vi "diffpsk.vi"() -> ()   [LabVIEW 2014]
panel:
  out "decoded\n data 2":bool[](array[boolean])
  out "demodulated output":dynamicdata(graph)
  out "Waveform DPSK":dynamicdata(graph)
  out "encoded data":bool[](array[boolean])
  in  "binary data":bool[](array[boolean])
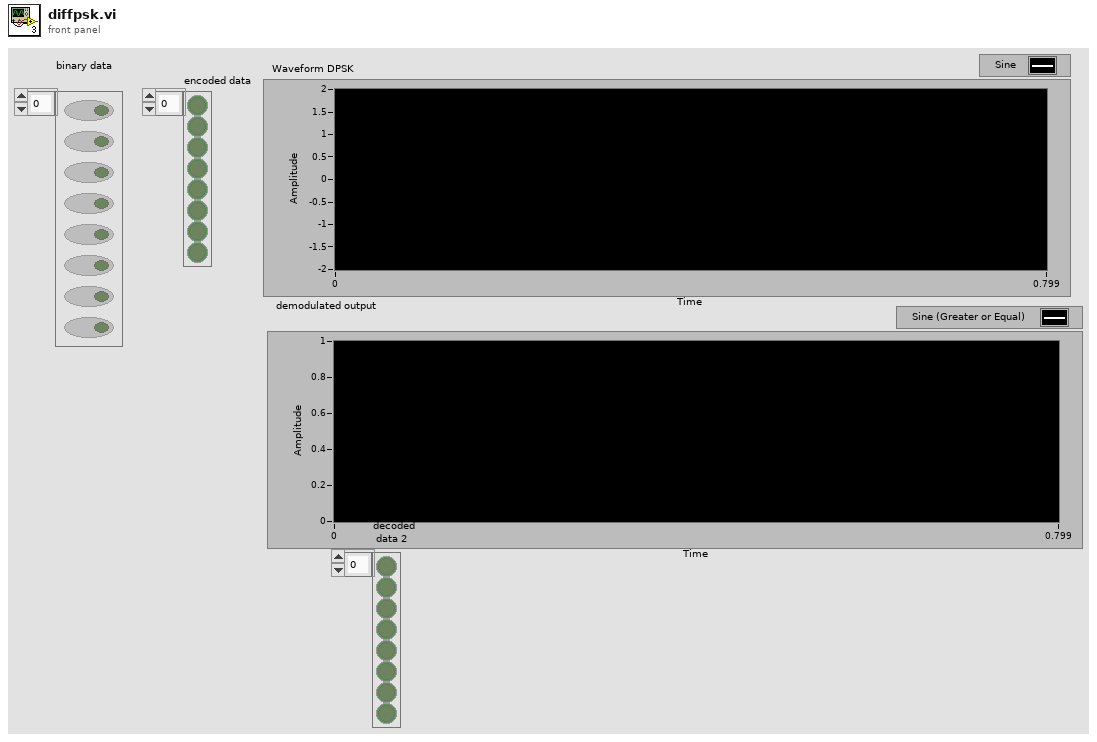
[diagram p1: front panel]
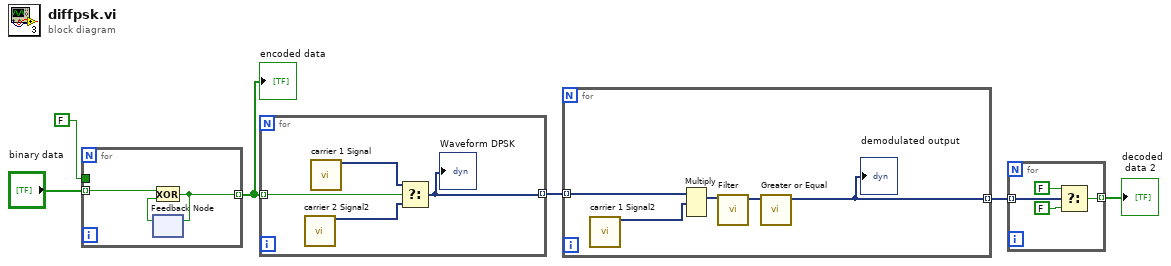
[diagram p0: block diagram]
diagram:
  n1 = for {
    tunnel: "binary data" -> [w9] mode=indexing
    tunnel: FALSE -> [_]
    tunnel: [w7] -> w4 mode=indexing
    n2 = feedback #1() -> (w8:bool)  [unwired: 1 in]
    n3 = Exclusive Or(1:w8, 2:w9) -> (0:w7:bool)
    n4 = feedback-in #1(w7) -> ()
  }
  "encoded data" <- w4
  n5 = for {
    tunnel: w4 -> [w11] mode=indexing
    tunnel: [w10] -> w3 mode=indexing
    n6 = call "carrier 2 Signal2"() -> ("Sine"=w12:dynamicdata)  [unwired: 14 in, 1 out]
    n7 = call "carrier 1 Signal"() -> ("Sine"=w13:dynamicdata)  [unwired: 14 in, 1 out]
    n8 = Select(t=w13, s=w11, f=w12) -> (s? t:f=w10:dynamicdata)
    "Waveform DPSK" <- w10
  }
  n9 = for {
    tunnel: w3 -> [w17] mode=indexing
    tunnel: [w14] -> w2 mode=indexing
    n10 = call "carrier 1 Signal2"() -> ("Sine"=w18:dynamicdata)  [unwired: 14 in, 1 out]
    n11 = Multiply(1:w18, 2:w17) -> (0:w16:dynamicdata)  [unwired: 1 in, 1 out]
    n12 = call "Filter"("Signal"=w16) -> ("Filtered Signal"=w15:dynamicdata)  [unwired: 9 in, 1 out]
    n13 = call "Greater or Equal"("Operand 1"=w15) -> ("Result"=w14:dynamicdata)  [unwired: 9 in, 1 out]
    "demodulated output" <- w14
  }
  n14 = for {
    tunnel: w2 -> [w20] mode=indexing
    tunnel: [w19] -> w1 mode=indexing
    n15 = Select(t=FALSE, s=w20, f=FALSE) -> (s? t:f=w19:bool)
  }
  "decoded\n data 2" <- w1
